vi "GT Get Control Info.vi"(8 "error in (no error)":errorcluster caption="错误输入（无错误）", 9 "pControlInfo":T1, 10 "control":i16, 11 "cardNum":i16) -> (0 "error out":errorcluster caption="错误输出", 1 "pControlInfo out":T1, 3 "function return":i16)   [LabVIEW 2020, in "gts1.lvlib"]
doc: "GT_API GT_GetControlInfo(short cardNum,short control,TControlInfo *pControlInfo);"
uses:
  gts1.lvlib
  dll/32bit/multi_card/gts.dll
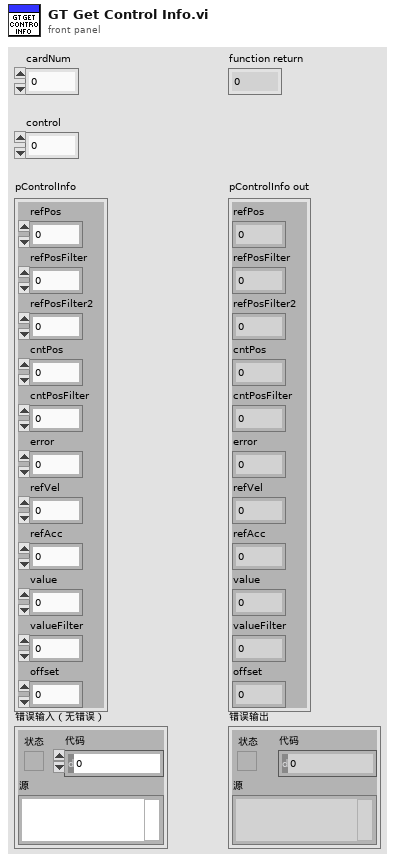
[diagram p1: front panel]
types:
  T1 = cluster{"refPos":dbl, "refPosFilter":dbl, "refPosFilter2":dbl, "cntPos":dbl, "cntPosFilter":dbl, "error":dbl, "refVel":dbl, "refAcc":dbl, "value":i16, "valueFilter":i16, "offset":i16}
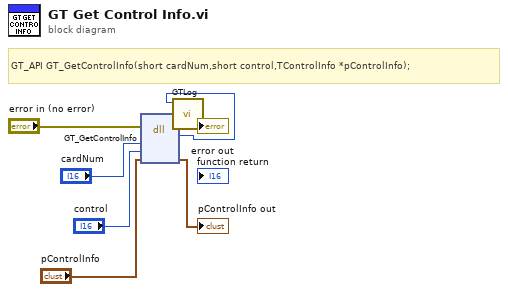
[diagram p0: block diagram]
diagram:
  # "GT_API GT_GetControlInfo(short cardNum,short control,TControlInfo *pControlInfo);"
  n1 = dll-call lib="C:/1228/dll/32bit/multi_card/gts.dll" fn="GT_GetControlInfo"(error in="error in (no error)", "cardNum"="cardNum", "control"="control", "pControlInfo"="pControlInfo") -> (error out=w3:errorcluster, w1:i16, "pControlInfo"=→"pControlInfo out":T1)  [unwired: 4 in, 1 out]
  n2 = call "GTLog.vi"("error in (no error)"=w3, "Numeric"=w1) -> ("error out"=→"error out":errorcluster)  [unwired: 9 in]
